vi "Network Stream Global Stop.vi"() -> ()   [LabVIEW 2023]
doc: "The global variable used to coordinate a stop between parallel loops in the Simple Network Streams example."
panel:
  in  "Target Stop":bool
  in  "Host Stop":bool
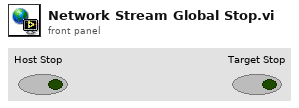
[diagram p1: front panel]
diagram:
